vi "hmp4000_core_global.vi"() -> ()   [LabVIEW 2022 SP3]
doc: "This Global variable contains driver's:\n- Attributes\n- Range Tables\n- Repeated Capabilities"
uses:
  type_Input_Format_Attribute.ctl
  type_Input_Format_RangeTable.ctl
  type_Input_Format_RepCap.ctl
  hmp4000_rsidr_core.lvlib
panel:
  in  "Repeated Capabilities":T1[](array[typedef])=[{"repCapName"="Channel", "indetifiers"=["CH1", "CH2", "CH3", "CH4"], "cmdValues"=["1", "2", "3", "4"]}]
  in  "Range Tables":T2[](array[typedef])=[{"Type"=2, "Name"="hmp4000_rngChannel", "Entries"=[{"Name"="Not Used", "Value 1"=0.0, "Value 2"=0.0, "Command"=""}, {"Name"="Channel 1", "Value 1"=1.0, "Value 2"=0.0, "Command"="1"}, {"Name"="Channel 2", "Value 1"=2.0, "Value 2"=0.0, "Command"="2"}, {"Name"="Channel 3", "Value 1"=3.0, "Value 2"=0.0, "Command"="3"}, {"Name"="Channel 4", "Value 1"=4.0, "Value 2"=0.0, "Command"="4"}]}, {"Type"=2, "Name"="hmp4000_rngMemoryIndex", "Entries"=[{"Name"="Index 1", "Value 1"=1.0, "Value 2"=0.0, "Command"="1"}, {"Name"="Index 2", "Value 1"=2.0, "Value 2"=0.0, "Command"="2"}, {"Name"="Index 3", "Value 1"=3.0, "Value 2"=0.0, "Command"="3"}]}, {"Type"=2, "Name"="hmp4000_rngOutput", "Entries"=[{"Name"="Channel 1", "Value 1"=1.0, "Value 2"=0.0, "Command"="OUTP1"}, {"Name"="Channel 2", "Value 1"=2.0, "Value 2"=0.0, "Command"="OUTP2"}, {"Name"="Channel 3", "Value 1"=3.0, "Value 2"=0.0, "Command"="OUTP3"}, {"Name"="Channel 4", "Value 1"=4.0, "Value 2"=0.0, "Command"="OUTP4"}]}, {"Type"=0, "Name"="hmp4000_rngOutputVoltage", "Entries"=[{"Name"="", "Value 1"=0.0, "Value 2"=32.0, "Command"=""}]}, {"Type"=0, "Name"="hmp4000_rngOutputCurrent", "Entries"=[{"Name"="", "Value 1"=0.0, "Value 2"=10.0, "Command"=""}]}, {"Type"=0, "Name"="hmp4000_rngMemoryLocation", "Entries"=[{"Name"="", "Value 1"=0.0, "Value 2"=9.0, "Command"=""}]}, {"Type"=0, "Name"="hmp4000_rngArbRepetition", "Entries"=[{"Name"="", "Value 1"=0.0, "Value 2"=255.0, "Command"=""}]}, {"Type"=0, "Name"="hmp4000_rngOVP", "Entries"=[{"Name"="", "Value 1"=0.0, "Value 2"=33.0, "Command"=""}]}, {"Type"=2, "Name"="hmp4000_rngBeeper", "Entries"=[{"Name"="Off", "Value 1"=0.0, "Value 2"=0.0, "Command"="OFF"}, {"Name"="On", "Value 1"=1.0, "Value 2"=0.0, "Command"="ON"}, {"Name"="Critical Event Only", "Value 1"=2.0, "Value 2"=0.0, "Command"="CRIT"}]}, {"Type"=2, "Name"="Hmp4000_rngOverVoltageProtectionMode", "Entries"=[{"Name"="Measured", "Value 1"=0.0, "Value 2"=0.0, "Command"="MEAS"}, {"Name"="Protected", "Value 1"=1.0, "Value 2"=0.0, "Command"="PROT"}]}] {"Type" items=["Range", "Coerced", "Discrete"]}
  in  "Attributes":T3[](array[typedef])=[{"Level"=1, "Class Only"=TRUE, "Identifier"="", "Descriptive Name"="Basic Operation", "Data Type"=4, "Command"="", "Access"=0, "Range Table"="", "Read Callback"="", "Write Callback"="", "Supported Models"="", "Instrument Options"="", "Flags"=0, "Help"="This class configures Basic Operation.\n\n(1) Selection Of Channel:\nThis attribute selects the channels. \n\n(2) Output State:\nThis attribute switches On or Off the output.\n\n(3) Settings Store Location:\nThis attribute stores the settings to selected locations of a nonvolatile memory.\n\n(4) Settings Recall Location:\nThis attribute recalls the settings from selected locations of a nonvolatile memory.\n\n(5) Beeper Mode:\nThis attribute configures the beeper."}, {"Level"=2, "Class Only"=FALSE, "Identifier"="HMP4000_ATTR_SELECTION_OF_CHANNEL", "Descriptive Name"="Selection Of Channel", "Data Type"=0, "Command"="INST:SEL", "Access"=2, "Range Table"="hmp4000_rngOutput", "Read Callback"="", "Write Callback"="", "Supported Models"="", "Instrument Options"="", "Flags"=0, "Help"="This attribute selects the channels.\n\nAvailable Repeated Capabilities:\nNone\n\nRemote-control command(s):\nINSTrument:SELect"}, {"Level"=2, "Class Only"=FALSE, "Identifier"="HMP4000_ATTR_OUTPUT_STATE", "Descriptive Name"="Output State", "Data Type"=3, "Command"="OUTP:STAT", "Access"=2, "Range Table"="", "Read Callback"="", "Write Callback"="", "Supported Models"="", "Instrument Options"="", "Flags"=0, "Help"="Turns the channel output ON or OFF. When switching the channel ON, General output switch is also switched ON. When switching the channel OFF, General output switch is not changed. If changing the General output switch status is not desired, use the HMP4000_ATTR_OUTPUT_SELECT.\n\nAvailable Repeated Capabilities:\nNone\n\nRemote-control command(s):\nOUTPut:STATe"}, {"Level"=2, "Class Only"=FALSE, "Identifier"="HMP4000_ATTR_GENERAL_OUTPUT_STATE", "Descriptive Name"="General Output State", "Data Type"=3, "Command"="OUTP:GEN", "Access"=2, "Range Table"="", "Read Callback"="", "Write Callback"="", "Supported Models"="", "Instrument Options"="", "Flags"=0, "Help"="Turning on / off all previous selected channels simultaneously.\n\nAvailable Repeated Capabilities:\nNone\n\nRemote-control command(s):\nOUTPut:GENeral"}, {"Level"=2, "Class Only"=FALSE, "Identifier"="HMP4000_ATTR_OUTPUT_SELECT", "Descriptive Name"="Output Select", "Data Type"=3, "Command"="OUTP:SEL", "Access"=2, "Range Table"="", "Read Callback"="", "Write Callback"="", "Supported Models"="", "Instrument Options"="", "Flags"=0, "Help"="Activates or deactivates the previous selected channel. If the channel is activated the channel LED lights up green in CV (constant voltage) mode or red in CC (constant current) mode.\n\nAvailable Repeated Capabilities:\nNone\n\nRemote-control command(s):\nOUTPut:SELect"}, {"Level"=2, "Class Only"=FALSE, "Identifier"="HMP4000_ATTR_SETTINGS_STORE_LOCATION", "Descriptive Name"="Settings Store Location", "Data Type"=0, "Command"="*SAV", "Access"=1, "Range Table"="hmp4000_rngMemoryLocation", "Read Callback"="", "Write Callback"="", "Supported Models"="", "Instrument Options"="", "Flags"=0, "Help"="This attribute stores the settings to selected locations of a nonvolatile memory.\n\nAvailable Repeated Capabilities:\nNone\n\nRemote-control command(s):\n*SAV"}, {"Level"=2, "Class Only"=FALSE, "Identifier"="HMP4000_ATTR_SETTINGS_RECALL_LOCATION", "Descriptive Name"="Settings Recall Location", "Data Type"=0, "Command"="*RCL", "Access"=1, "Range Table"="hmp4000_rngMemoryLocation", "Read Callback"="", "Write Callback"="", "Supported Models"="", "Instrument Options"="", "Flags"=0, "Help"="This attribute recalls the settings from selected locations of a nonvolatile memory.\n\nAvailable Repeated Capabilities:\nNone\n\nRemote-control command(s):\n*RCL"}, {"Level"=2, "Class Only"=FALSE, "Identifier"="HMP4000_ATTR_BEEPER_MODE", "Descriptive Name"="Beeper Mode", "Data Type"=0, "Command"="SYST:BEEP:IMM", "Access"=2, "Range Table"="hmp4000_rngBeeper", "Read Callback"="", "Write Callback"="", "Supported Models"="", "Instrument Options"="", "Flags"=0, "Help"="This attribute configures the beeper.\n\nAvailable Repeated Capabilities:\nNone\n\nRemote-control command(s):\nSYSTem:BEEPer:IMMediate"}, {"Level"=1, "Class Only"=TRUE, "Identifier"="", "Descriptive Name"="Voltage and Current", "Data Type"=4, "Command"="", "Access"=0, "Range Table"="", "Read Callback"="", "Write Callback"="", "Supported Models"="", "Instrument Options"="", "Flags"=0, "Help"="This class configures Voltage and Current.\n\n(1) Output Voltage Level:\nThis attribute adjusts the output voltage level. \n\n(2) Output Voltage Level Step:\nThis attribute configures the output voltage step value. \n\n(3) Over Voltage Protection Level:\nThis attribute configures the over voltage protection (OVP). \n\n(4) Query Over Voltage Protection Status:\nThis attribute queries the over voltage protection (OVP) status. \n\n(5) Over Voltage Protection Clear:\nThis attribute clears the over voltage protection (OVP). \n\n(6) Output Current Level:\nThis attribute adjusts the output current level. \n\n(7) Output Current Level Step:\nThis attribute configures the output current step value. \n\n(8) Electronic Fuse State:\nThis attribute switches On or Off the electronic fuse.\n\n(9) Query Electronic Fuse Status:\nThis attribute queries the electronic fuse status. \n\n(10) Electronic Fuse Channel Link:\nThis attribute link electronic fuse to the channel.\n\n(11) Electronic Fuse Channel Unlink:\nThis attribute unlink electronic fuse from the channel."}, {"Level"=2, "Class Only"=FALSE, "Identifier"="HMP4000_ATTR_OUTPUT_VOLTAGE_LEVEL", "Descriptive Name"="Output Voltage Level", "Data Type"=1, "Command"="SOUR:VOLT:LEV:AMPL", "Access"=2, "Range Table"="hmp4000_rngOutputVoltage", "Read Callback"="", "Write Callback"="", "Supported Models"="", "Instrument Options"="", "Flags"=0, "Help"="This attribute adjusts the output voltage level.\n\nAvailable Repeated Capabilities:\nNone\n\nRemote-control command(s):\nSOURce:VOLTage:LEVel:AMPLitude"}, {"Level"=2, "Class Only"=FALSE, "Identifier"="HMP4000_ATTR_OUTPUT_VOLTAGE_LEVEL_MAX", "Descriptive Name"="Output Voltage Level Max", "Data Type"=1, "Command"="VOLT? MAX", "Access"=0, "Range Table"="", "Read Callback"="", "Write Callback"="", "Supported Models"="", "Instrument Options"="", "Flags"=0, "Help"="Queires the maximum available output voltage.\n\nAvailable Repeated Capabilities:\nNone\n\nRemote-control command(s):\n[SOURce:]VOLTage[:LEVel][:IMMediate][:AMPLitude]"}, {"Level"=2, "Class Only"=FALSE, "Identifier"="HMP4000_ATTR_OUTPUT_VOLTAGE_LEVEL_STEP", "Descriptive Name"="Output Voltage Level Step", "Data Type"=1, "Command"="SOUR:VOLT:LEV:AMPL:STEP:INCR", "Access"=2, "Range Table"="hmp4000_rngOutputVoltage", "Read Callback"="", "Write Callback"="", "Supported Models"="", "Instrument Options"="", "Flags"=0, "Help"="This attribute configures the output voltage step value.\n\nAvailable Repeated Capabilities:\nNone\n\nRemote-control command(s):\nSOURce:VOLTage:LEVel:AMPLitude:STEP:INCRement"}, {"Level"=2, "Class Only"=FALSE, "Identifier"="HMP4000_ATTR_OVER_VOLTAGE_PROTECTION_LEVEL", "Descriptive Name"="Over Voltage Protection Level", "Data Type"=1, "Command"="VOLT:PROT:LEV", "Access"=2, "Range Table"="hmp4000_rngOVP", "Read Callback"="", "Write Callback"="", "Supported Models"="", "Instrument Options"="", "Flags"=0, "Help"="This attribute configures the over voltage protection (OVP).\n\nAvailable Repeated Capabilities:\nNone\n\nRemote-control command(s):\nVOLTage:PROTection:LEVel"}, {"Level"=2, "Class Only"=FALSE, "Identifier"="HMP4000_ATTR_QUERY_OVER_VOLTAGE_PROTECTION_STATUS", "Descriptive Name"="Query Over Voltage Protection Status", "Data Type"=3, "Command"="VOLT:PROT:TRIP?", "Access"=0, "Range Table"="", "Read Callback"="", "Write Callback"="", "Supported Models"="", "Instrument Options"="", "Flags"=0, "Help"="This attribute queries the over voltage protection (OVP) status.\n\nAvailable Repeated Capabilities:\nNone\n\nRemote-control command(s):\nVOLTage:PROTection:TRIPped?"}, {"Level"=2, "Class Only"=FALSE, "Identifier"="HMP4000_ATTR_OVER_VOLTAGE_PROTECTION_CLEAR", "Descriptive Name"="Over Voltage Protection Clear", "Data Type"=4, "Command"="VOLT:PROT:CLE", "Access"=1, "Range Table"="", "Read Callback"="", "Write Callback"="", "Supported Models"="", "Instrument Options"="", "Flags"=0, "Help"="This attribute clears the over voltage protection (OVP).\n\nAvailable Repeated Capabilities:\nNone\n\nRemote-control command(s):\nVOLTage:PROTection:CLEar"}, {"Level"=2, "Class Only"=FALSE, "Identifier"="HMP4000_ATTR_OVER_VOLTAGE_PROTECTION_MODE", "Descriptive Name"="Over Voltage Protection Mode", "Data Type"=0, "Command"="VOLT:PROT:MODE", "Access"=2, "Range Table"="Hmp4000_rngOverVoltageProtectionMode", "Read Callback"="", "Write Callback"="", "Supported Models"="", "Instrument Options"="", "Flags"=0, "Help"="Sets the OVP mode for the previously selected channel.\n\nAvailable Repeated Capabilities:\nNone\n\nRemote-control command(s):\n[SOURce:]VOLTage:PROTection:MODE"}, {"Level"=2, "Class Only"=FALSE, "Identifier"="HMP4000_ATTR_OUTPUT_CURRENT_LEVEL", "Descriptive Name"="Output Current Level", "Data Type"=1, "Command"="SOUR:CURR:LEV:AMPL", "Access"=2, "Range Table"="hmp4000_rngOutputCurrent", "Read Callback"="", "Write Callback"="", "Supported Models"="", "Instrument Options"="", "Flags"=0, "Help"="This attribute adjusts the output current level.\n\nAvailable Repeated Capabilities:\nNone\n\nRemote-control command(s):\nSOURce:CURRent:LEVel:AMPLitude"}, {"Level"=2, "Class Only"=FALSE, "Identifier"="HMP4000_ATTR_OUTPUT_CURRENT_LEVEL_MAX", "Descriptive Name"="Output Current Level Max", "Data Type"=1, "Command"="CURR? MAX", "Access"=0, "Range Table"="", "Read Callback"="", "Write Callback"="", "Supported Models"="", "Instrument Options"="", "Flags"=0, "Help"="Queries the maximum allowed current value.\n\nAvailable Repeated Capabilities:\nNone\n\nRemote-control command(s):\n[SOURce:]CURRent[:LEVel][:IMMediate][:AMPLitude]"}, {"Level"=2, "Class Only"=FALSE, "Identifier"="HMP4000_ATTR_OUTPUT_CURRENT_LEVEL_STEP", "Descriptive Name"="Output Current Level Step", "Data Type"=1, "Command"="SOUR:CURR:LEV:AMPL:STEP:INCR", "Access"=2, "Range Table"="hmp4000_rngOutputCurrent", "Read Callback"="", "Write Callback"="", "Supported Models"="", "Instrument Options"="", "Flags"=0, "Help"="This attribute configures the output current step value.\n\nAvailable Repeated Capabilities:\nNone\n\nRemote-control command(s):\nSOURce:CURRent:LEVel:AMPLitude:STEP:INCRement"}, {"Level"=2, "Class Only"=FALSE, "Identifier"="HMP4000_ATTR_ELECTRONIC_FUSE_STATE", "Descriptive Name"="Electronic Fuse State", "Data Type"=3, "Command"="FUSE:STAT", "Access"=2, "Range Table"="", "Read Callback"="", "Write Callback"="", "Supported Models"="", "Instrument Options"="", "Flags"=0, "Help"="This attribute switches On or Off the electronic fuse.\n\nAvailable Repeated Capabilities:\nNone\n\nRemote-control command(s):\nFUSE:STATe"}, {"Level"=2, "Class Only"=FALSE, "Identifier"="HMP4000_ATTR_QUERY_ELECTRONIC_FUSE_STATUS", "Descriptive Name"="Query Electronic Fuse Status", "Data Type"=3, "Command"="FUSE:TRIP?", "Access"=0, "Range Table"="", "Read Callback"="", "Write Callback"="", "Supported Models"="", "Instrument Options"="", "Flags"=0, "Help"="This attribute queries the electronic fuse status.\n\nAvailable Repeated Capabilities:\nNone\n\nRemote-control command(s):\nFUSE:TRIPped?"}, {"Level"=2, "Class Only"=FALSE, "Identifier"="HMP4000_ATTR_ELECTRONIC_FUSE_CHANNEL_LINK", "Descriptive Name"="Electronic Fuse Channel Link", "Data Type"=0, "Command"="FUSE:LINK", "Access"=1, "Range Table"="hmp4000_rngChannel", "Read Callback"="", "Write Callback"="", "Supported Models"="", "Instrument Options"="", "Flags"=0, "Help"="This attribute link electronic fuse to the channel.\n\nAvailable Repeated Capabilities:\nNone\n\nRemote-control command(s):\nFUSE:LINK"}, {"Level"=2, "Class Only"=FALSE, "Identifier"="HMP4000_ATTR_ELECTRONIC_FUSE_CHANNEL_UNLINK", "Descriptive Name"="Electronic Fuse Channel Unlink", "Data Type"=0, "Command"="FUSE:UNL", "Access"=1, "Range Table"="hmp4000_rngChannel", "Read Callback"="", "Write Callback"="", "Supported Models"="", "Instrument Options"="", "Flags"=0, "Help"="This attribute unlink electronic fuse from the channel.\n\nAvailable Repeated Capabilities:\nNone\n\nRemote-control command(s):\nFUSE:UNLink"}, {"Level"=2, "Class Only"=TRUE, "Identifier"="", "Descriptive Name"="Query Combined Voltage And Current", "Data Type"=4, "Command"="", "Access"=0, "Range Table"="", "Read Callback"="", "Write Callback"="", "Supported Models"="", "Instrument Options"="", "Flags"=0, "Help"="This function queries combined setting of voltage and current. \n\nFirst result is Voltage Value, second is Current.\n\nRemote-control command(s):\nAPPLy?"}, {"Level"=1, "Class Only"=TRUE, "Identifier"="", "Descriptive Name"="Arbitrary Generator", "Data Type"=4, "Command"="", "Access"=0, "Range Table"="", "Read Callback"="", "Write Callback"="", "Supported Models"="", "Instrument Options"="", "Flags"=0, "Help"="This class configures Arbitrary Generator.\n\n(1) Arbitrary Generator Repetition:\nNo. of repetition. The maximum number of repetitions is 255. If 0 is selected, the waveform will be repeated indefi nitely.\n\n(2) Arbitrary Generator Start Channel:\nThis attribute selects the channel for starting arbitrary generator. \n\n(3) Arbitrary Generator Stop Channel:\nThis attribute selects the channel for stoping arbitrary generator. \n\n(4) Arbitrary Generator Data Transfer Channel:\nThis attribute selects the channel where the data entered are sent to.\n\n(5) Arbitrary Generator Save:\nThis attribute selects the storage for saving arbitrary generator waveform data. \n\n\n(6) Arbitrary Generator Recall:\nThis attribute selects the storage for recalling arbitrary generator waveform data. \n\n(7) Arbitrary Generator Clear:\nThis attribute selects the storage for clearing arbitrary generator waveform data."}, {"Level"=2, "Class Only"=TRUE, "Identifier"="", "Descriptive Name"="Configure Arbitrary Generator Waveform Data", "Data Type"=4, "Command"="", "Access"=0, "Range Table"="", "Read Callback"="", "Write Callback"="", "Supported Models"="", "Instrument Options"="", "Flags"=0, "Help"="This function sets the parameters of the freely programmable waveforms. Set points defining voltage, current and dwell\ntime are required.\n\nA maximum of 128 set points (index 0 ... 128) may be used and\nwill be repetitively addressed.\n\nThe maximum number of repetitions is 255. If Repetitons 0 is selected, the waveform will be repeated indefinitely. \n\nRemote-control command(s):\nARBitrary:DATA <voltage1, current1, time1, voltage2, ...>"}, {"Level"=2, "Class Only"=FALSE, "Identifier"="HMP4000_ATTR_ARBITRARY_GENERATOR_REPETITION", "Descriptive Name"="Arbitrary Generator Repetition", "Data Type"=0, "Command"="ARB:REP", "Access"=2, "Range Table"="hmp4000_rngArbRepetition", "Read Callback"="", "Write Callback"="", "Supported Models"="", "Instrument Options"="", "Flags"=0, "Help"="No. of repetition. The maximum number of repetitions is 255. If 0 is selected, the waveform will be repeated indefi nitely.\n\nAvailable Repeated Capabilities:\nNone\n\nRemote-control command(s):\nARBitrary:REPetitions"}, {"Level"=2, "Class Only"=FALSE, "Identifier"="HMP4000_ATTR_ARBITRARY_GENERATOR_START_CHANNEL", "Descriptive Name"="Arbitrary Generator Start Channel", "Data Type"=0, "Command"="ARB:STAR", "Access"=1, "Range Table"="hmp4000_rngChannel", "Read Callback"="", "Write Callback"="", "Supported Models"="", "Instrument Options"="", "Flags"=0, "Help"="This attribute selects the channel for starting arbitrary generator.\n\nAvailable Repeated Capabilities:\nNone\n\nRemote-control command(s):\nARBitrary:STARt"}, {"Level"=2, "Class Only"=FALSE, "Identifier"="HMP4000_ATTR_ARBITRARY_GENERATOR_STOP_CHANNEL", "Descriptive Name"="Arbitrary Generator Stop Channel", "Data Type"=0, "Command"="ARB:STOP", "Access"=1, "Range Table"="hmp4000_rngChannel", "Read Callback"="", "Write Callback"="", "Supported Models"="", "Instrument Options"="", "Flags"=0, "Help"="This attribute selects the channel for stoping arbitrary generator.\n\nAvailable Repeated Capabilities:\nNone\n\nRemote-control command(s):\nARBitrary:STOP"}, {"Level"=2, "Class Only"=FALSE, "Identifier"="HMP4000_ATTR_ARBITRARY_GENERATOR_DATA_TRANSFER_CHANNEL", "Descriptive Name"="Arbitrary Generator Data Transfer Channel", "Data Type"=0, "Command"="ARB:TRAN", "Access"=1, "Range Table"="hmp4000_rngChannel", "Read Callback"="", "Write Callback"="", "Supported Models"="", "Instrument Options"="", "Flags"=0, "Help"="This attribute selects the channel where the data entered are sent to.\n\nAvailable Repeated Capabilities:\nNone\n\nRemote-control command(s):\nARBitrary:TRANsfer"}, {"Level"=2, "Class Only"=FALSE, "Identifier"="HMP4000_ATTR_ARBITRARY_GENERATOR_SAVE", "Descriptive Name"="Arbitrary Generator Save", "Data Type"=0, "Command"="ARB:SAVE", "Access"=1, "Range Table"="hmp4000_rngMemoryIndex", "Read Callback"="", "Write Callback"="hmp4000_Delayed_Int32_WriteCallback.vi", "Supported Models"="", "Instrument Options"="", "Flags"=0, "Help"="This attribute selects the storage for saving arbitrary generator waveform data.\n\nAvailable Repeated Capabilities:\nNone\n\nRemote-control command(s):\nARBitrary:SAVE"}, {"Level"=2, "Class Only"=FALSE, "Identifier"="HMP4000_ATTR_ARBITRARY_GENERATOR_RECALL", "Descriptive Name"="Arbitrary Generator Recall", "Data Type"=0, "Command"="ARB:REST", "Access"=1, "Range Table"="hmp4000_rngMemoryIndex", "Read Callback"="", "Write Callback"="", "Supported Models"="", "Instrument Options"="", "Flags"=0, "Help"="This attribute selects the storage for recalling arbitrary generator waveform data.\n\nAvailable Repeated Capabilities:\nNone\n\nRemote-control command(s):\nARBitrary:RESTore"}, {"Level"=2, "Class Only"=FALSE, "Identifier"="HMP4000_ATTR_ARBITRARY_GENERATOR_CLEAR", "Descriptive Name"="Arbitrary Generator Clear", "Data Type"=0, "Command"="ARB:CLE", "Access"=1, "Range Table"="hmp4000_rngMemoryIndex", "Read Callback"="", "Write Callback"="", "Supported Models"="", "Instrument Options"="", "Flags"=0, "Help"="This attribute selects the storage for clearing arbitrary generator waveform data.\n\nAvailable Repeated Capabilities:\nNone\n\nRemote-control command(s):\nARBitrary:CLEar"}, {"Level"=1, "Class Only"=TRUE, "Identifier"="", "Descriptive Name"="Measurement", "Data Type"=4, "Command"="", "Access"=0, "Range Table"="", "Read Callback"="", "Write Callback"="", "Supported Models"="", "Instrument Options"="", "Flags"=0, "Help"="This class queries measurement.\n\n(1) Measurement DC Voltage:\nThis attribute queries the measured voltage value. \n\n(2) Measurement DC Current:\nThis attribute queries the measured Current value."}, {"Level"=2, "Class Only"=FALSE, "Identifier"="HMP4000_ATTR_MEASUREMENT_DC_VOLTAGE", "Descriptive Name"="Measurement DC Voltage", "Data Type"=1, "Command"="MEAS:VOLT:DC?", "Access"=0, "Range Table"="", "Read Callback"="", "Write Callback"="", "Supported Models"="", "Instrument Options"="", "Flags"=0, "Help"="This attribute queries the measured voltage value.\n\nAvailable Repeated Capabilities:\nNone\n\nRemote-control command(s):\nMEASure:VOLTage:DC?"}, {"Level"=2, "Class Only"=FALSE, "Identifier"="HMP4000_ATTR_MEASUREMENT_DC_CURRENT", "Descriptive Name"="Measurement DC Current", "Data Type"=1, "Command"="MEAS:CURR:DC?", "Access"=0, "Range Table"="", "Read Callback"="", "Write Callback"="", "Supported Models"="", "Instrument Options"="", "Flags"=0, "Help"="This attribute queries the measured Current value.\n\nAvailable Repeated Capabilities:\nNone\n\nRemote-control command(s):\nMEASure:CURRent:DC?"}, {"Level"=1, "Class Only"=TRUE, "Identifier"="", "Descriptive Name"="Utility Functions", "Data Type"=4, "Command"="", "Access"=0, "Range Table"="", "Read Callback"="", "Write Callback"="", "Supported Models"="", "Instrument Options"="", "Flags"=0, "Help"="Various utility attributes.\n\n(1) System Version:\nGets system version.\n\n(2) System Error:\nThis attribute queries the earliest entry in the error queue, and deletes it after the readout.\n\n(3) System All Errors:\nReads all errors from instrument.\n\n(4) Questionable Enable Register:\nThis attribute configures the selected register enable values.\n\n(5) Questionable Instrument Enable Register:\nThis attribute configures the selected register enable values.\n\n(6) Questionable Instrument Specific Enable Register:\nThis attribute configures the selected register enable values.\n\n(7) Questionable Instrument Specific Condition Register:\nThis attribute queries the selected register condition values."}, {"Level"=2, "Class Only"=TRUE, "Identifier"="", "Descriptive Name"="Add Stream Logger", "Data Type"=4, "Command"="", "Access"=0, "Range Table"="", "Read Callback"="", "Write Callback"="", "Supported Models"="", "Instrument Options"="", "Flags"=0, "Help"="This method adds the stream for logging."}, {"Level"=2, "Class Only"=TRUE, "Identifier"="", "Descriptive Name"="Remove Stream Logger", "Data Type"=4, "Command"="", "Access"=0, "Range Table"="", "Read Callback"="", "Write Callback"="", "Supported Models"="", "Instrument Options"="", "Flags"=0, "Help"="This method removes the stream for logging."}, {"Level"=2, "Class Only"=TRUE, "Identifier"="", "Descriptive Name"="Write String To Log", "Data Type"=4, "Command"="", "Access"=0, "Range Table"="", "Read Callback"="", "Write Callback"="", "Supported Models"="", "Instrument Options"="", "Flags"=0, "Help"="Writes string message to log."}, {"Level"=2, "Class Only"=TRUE, "Identifier"="", "Descriptive Name"="Read To File From Instrument", "Data Type"=4, "Command"="", "Access"=0, "Range Table"="", "Read Callback"="", "Write Callback"="", "Supported Models"="", "Instrument Options"="", "Flags"=0, "Help"="Is used to read data from the instrument and write it to a user specified file on the host computer.\n\nRemote-control command(s):\nMMEMory:DATA? <file_name>"}, {"Level"=2, "Class Only"=TRUE, "Identifier"="", "Descriptive Name"="Write From File To Instrument", "Data Type"=4, "Command"="", "Access"=0, "Range Table"="", "Read Callback"="", "Write Callback"="", "Supported Models"="", "Instrument Options"="", "Flags"=0, "Help"="Is used to read data from the host computer and write it to a user specified file in the instrument.\n\nRemote-control command(s):\nMMEMory:DATA <file_name>"}, {"Level"=2, "Class Only"=TRUE, "Identifier"="", "Descriptive Name"="Query Binary Data Block To Stream", "Data Type"=4, "Command"="", "Access"=0, "Range Table"="", "Read Callback"="", "Write Callback"="", "Supported Models"="", "Instrument Options"="", "Flags"=0, "Help"="Queries IEEE binary data block from instrument to stream. Use it for fast fetching of binary block data."}, {"Level"=2, "Class Only"=TRUE, "Identifier"="", "Descriptive Name"="Query Binary Data Block To Stream With OPC", "Data Type"=4, "Command"="", "Access"=0, "Range Table"="", "Read Callback"="", "Write Callback"="", "Supported Models"="", "Instrument Options"="", "Flags"=0, "Help"="Queries IEEE binary data block from instrument to stream. Use it for fast fetching of binary block data. If timeout is null, -1 or 0, the current Opc Timeout is used."}, {"Level"=2, "Class Only"=TRUE, "Identifier"="", "Descriptive Name"="Write Binary Block From Stream", "Data Type"=4, "Command"="", "Access"=0, "Range Table"="", "Read Callback"="", "Write Callback"="", "Supported Models"="", "Instrument Options"="", "Flags"=0, "Help"="Writes IEEE binary data block from stream to instrument. You need to specify the SCPI command to prepend the binary data block."}, {"Level"=2, "Class Only"=TRUE, "Identifier"="", "Descriptive Name"="Query Bool", "Data Type"=4, "Command"="", "Access"=0, "Range Table"="", "Read Callback"="", "Write Callback"="", "Supported Models"="", "Instrument Options"="", "Flags"=0, "Help"="This method queries the bool value."}, {"Level"=2, "Class Only"=TRUE, "Identifier"="", "Descriptive Name"="Query Int32", "Data Type"=4, "Command"="", "Access"=0, "Range Table"="", "Read Callback"="", "Write Callback"="", "Supported Models"="", "Instrument Options"="", "Flags"=0, "Help"="This method queries the int32 value."}, {"Level"=2, "Class Only"=TRUE, "Identifier"="", "Descriptive Name"="Query Double", "Data Type"=4, "Command"="", "Access"=0, "Range Table"="", "Read Callback"="", "Write Callback"="", "Supported Models"="", "Instrument Options"="", "Flags"=0, "Help"="This method queries the double value."}, {"Level"=2, "Class Only"=TRUE, "Identifier"="", "Descriptive Name"="Query String", "Data Type"=4, "Command"="", "Access"=0, "Range Table"="", "Read Callback"="", "Write Callback"="", "Supported Models"="", "Instrument Options"="", "Flags"=0, "Help"="This method queries the string value."}, {"Level"=2, "Class Only"=TRUE, "Identifier"="", "Descriptive Name"="Write Command with OPC sync", "Data Type"=4, "Command"="", "Access"=0, "Range Table"="", "Read Callback"="", "Write Callback"="", "Supported Models"="", "Instrument Options"="", "Flags"=0, "Help"="Sends a command to the instrument synchronised with OPC-polling. Use this function to wait for an instrument operation that can take a long time to complete, e.g. self-alignment. If timeout is null, -1 or 0, the current Opc Timeout is used."}, {"Level"=2, "Class Only"=TRUE, "Identifier"="", "Descriptive Name"="Query with OPC sync", "Data Type"=4, "Command"="", "Access"=0, "Range Table"="", "Read Callback"="", "Write Callback"="", "Supported Models"="", "Instrument Options"="", "Flags"=0, "Help"="Sends a query to the instrument synchronised with OPC-polling. Use this function to wait for a response that can take a long time to complete e.g. self-alignment, calibration or self-test. If timeout is null, -1 or 0, the current Opc Timeout is used."}, {"Level"=2, "Class Only"=TRUE, "Identifier"="", "Descriptive Name"="Self Test", "Data Type"=4, "Command"="", "Access"=0, "Range Table"="", "Read Callback"="", "Write Callback"="", "Supported Models"="", "Instrument Options"="", "Flags"=0, "Help"="Runs the instrument's self test routine."}, {"Level"=2, "Class Only"=TRUE, "Identifier"="", "Descriptive Name"="Revision Query", "Data Type"=4, "Command"="", "Access"=0, "Range Table"="", "Read Callback"="", "Write Callback"="", "Supported Models"="", "Instrument Options"="", "Flags"=0, "Help"="Returns the revision numbers of the instrument driver and instrument firmware, and tells the user with which  instrument firmware this revision of the driver is compatible."}, {"Level"=2, "Class Only"=TRUE, "Identifier"="", "Descriptive Name"="Delay", "Data Type"=4, "Command"="", "Access"=0, "Range Table"="", "Read Callback"="", "Write Callback"="", "Supported Models"="", "Instrument Options"="", "Flags"=0, "Help"="Suspends the program for the selected number of second."}, {"Level"=2, "Class Only"=TRUE, "Identifier"="", "Descriptive Name"="Error Query All", "Data Type"=4, "Command"="", "Access"=0, "Range Table"="", "Read Callback"="", "Write Callback"="", "Supported Models"="", "Instrument Options"="", "Flags"=0, "Help"="Returns all error.\n\nRemote-control command(s):\nSYSTem:ERRor?"}, {"Level"=2, "Class Only"=TRUE, "Identifier"="", "Descriptive Name"="Get Instrument Options", "Data Type"=4, "Command"="", "Access"=0, "Range Table"="", "Read Callback"="", "Write Callback"="", "Supported Models"="", "Instrument Options"="", "Flags"=0, "Help"="Returns all the instrument options.\n\nRemote-control command(s):\n*OPT?"}, {"Level"=2, "Class Only"=TRUE, "Identifier"="", "Descriptive Name"="Read Bytes", "Data Type"=4, "Command"="", "Access"=0, "Range Table"="", "Read Callback"="", "Write Callback"="", "Supported Models"="", "Instrument Options"="", "Flags"=0, "Help"="Reads a complete response from the instrument."}, {"Level"=2, "Class Only"=TRUE, "Identifier"="", "Descriptive Name"="Read String", "Data Type"=4, "Command"="", "Access"=0, "Range Table"="", "Read Callback"="", "Write Callback"="", "Supported Models"="", "Instrument Options"="", "Flags"=0, "Help"="Reads a complete response from the instrument and returns it as a string."}, {"Level"=2, "Class Only"=TRUE, "Identifier"="", "Descriptive Name"="Write Bytes", "Data Type"=4, "Command"="", "Access"=0, "Range Table"="", "Read Callback"="", "Write Callback"="", "Supported Models"="", "Instrument Options"="", "Flags"=0, "Help"="Write an array of bytes to the device."}, {"Level"=2, "Class Only"=TRUE, "Identifier"="", "Descriptive Name"="Write String", "Data Type"=4, "Command"="", "Access"=0, "Range Table"="", "Read Callback"="", "Write Callback"="", "Supported Models"="", "Instrument Options"="", "Flags"=0, "Help"="Write a string to the device."}, {"Level"=2, "Class Only"=FALSE, "Identifier"="HMP4000_ATTR_SYSTEM_VERSION", "Descriptive Name"="System Version", "Data Type"=2, "Command"="SYST:VERSion?", "Access"=0, "Range Table"="", "Read Callback"="", "Write Callback"="", "Supported Models"="", "Instrument Options"="", "Flags"=0, "Help"="Gets system version.\n\nAvailable Repeated Capabilities:\nNone\n\nRemote-control command(s):\nSYSTem:VERSion?"}, {"Level"=2, "Class Only"=FALSE, "Identifier"="HMP4000_ATTR_SYSTEM_ERROR", "Descriptive Name"="System Error", "Data Type"=2, "Command"="SYST:ERRor?", "Access"=0, "Range Table"="", "Read Callback"="", "Write Callback"="", "Supported Models"="", "Instrument Options"="", "Flags"=0, "Help"="This attribute queries the earliest entry in the error queue, and deletes it after the readout.\n\nAvailable Repeated Capabilities:\nNone\n\nRemote-control command(s):\nSYSTem:ERRor?"}, {"Level"=2, "Class Only"=FALSE, "Identifier"="HMP4000_ATTR_SYSTEM_ALL_ERRORS", "Descriptive Name"="System All Errors", "Data Type"=2, "Command"="SYST:ERR:ALL?", "Access"=0, "Range Table"="", "Read Callback"="", "Write Callback"="", "Supported Models"="", "Instrument Options"="", "Flags"=0, "Help"="Reads all errors from instrument.\n\nAvailable Repeated Capabilities:\nNone\n\nRemote-control command(s):\nSYSTem:ERRor:ALL?"}, {"Level"=2, "Class Only"=FALSE, "Identifier"="HMP4000_ATTR_SYSTEM_LOCAL", "Descriptive Name"="System Local", "Data Type"=4, "Command"="SYST:LOC", "Access"=1, "Range Table"="", "Read Callback"="", "Write Callback"="", "Supported Models"="", "Instrument Options"="", "Flags"=2, "Help"="Sets the system to front panel control. The front panel control is unlocked.\n\nAvailable Repeated Capabilities:\nNone\n\nRemote-control command(s):\nSYSTem:LOCal"}, {"Level"=2, "Class Only"=FALSE, "Identifier"="HMP4000_ATTR_SYSTEM_REMOTE", "Descriptive Name"="System Remote", "Data Type"=4, "Command"="SYST:REM", "Access"=1, "Range Table"="", "Read Callback"="", "Write Callback"="", "Supported Models"="", "Instrument Options"="", "Flags"=2, "Help"="Sets the system to remote state. The front panel control is locked. By pushing the REMOTE button the front panel control will be activated. If the instrument receives a remote command it will be switched into remote control automatically (REMOTE button LED lights up).\n\nAvailable Repeated Capabilities:\nNone\n\nRemote-control command(s):\nSYSTem:REMote"}, {"Level"=2, "Class Only"=FALSE, "Identifier"="HMP4000_ATTR_SYSTEM_REMOTE_LOCK", "Descriptive Name"="System Remote Lock", "Data Type"=4, "Command"="SYST:RWL", "Access"=1, "Range Table"="", "Read Callback"="", "Write Callback"="", "Supported Models"="", "Instrument Options"="", "Flags"=2, "Help"="Sets the system to remote state. The front panel control is locked and can not be unlocked via REMOTE button). You are only able to unlock the front panel control via SCPI command SYSTem:LOCal.\n\nAvailable Repeated Capabilities:\nNone\n\nRemote-control command(s):\nSYSTem:RWLock"}, {"Level"=2, "Class Only"=FALSE, "Identifier"="HMP4000_ATTR_SYSTEM_REMOTE_MIX", "Descriptive Name"="System Remote Mix", "Data Type"=4, "Command"="SYST:MIX", "Access"=1, "Range Table"="", "Read Callback"="", "Write Callback"="", "Supported Models"="", "Instrument Options"="", "Flags"=2, "Help"="Sets the system to remote state. The front panel and remote control are possible simultaneously (mixed mode).\n\nAvailable Repeated Capabilities:\nNone\n\nRemote-control command(s):\nSYSTem:MIX"}, {"Level"=2, "Class Only"=FALSE, "Identifier"="HMP4000_ATTR_QUESTIONABLE_ENABLE_REGISTER", "Descriptive Name"="Questionable Enable Register", "Data Type"=0, "Command"="STAT:QUES:ENAB", "Access"=2, "Range Table"="", "Read Callback"="", "Write Callback"="", "Supported Models"="", "Instrument Options"="", "Flags"=0, "Help"="This attribute configures the selected register enable values.\n\nAvailable Repeated Capabilities:\nNone\n\nRemote-control command(s):\nSTATus:QUEStionable:ENABle"}, {"Level"=2, "Class Only"=FALSE, "Identifier"="HMP4000_ATTR_QUESTIONABLE_INSTRUMENT_ENABLE_REGISTER", "Descriptive Name"="Questionable Instrument Enable Register", "Data Type"=0, "Command"="STAT:QUES:INST:ENAB", "Access"=2, "Range Table"="", "Read Callback"="", "Write Callback"="", "Supported Models"="", "Instrument Options"="", "Flags"=0, "Help"="This attribute configures the selected register enable values.\n\nAvailable Repeated Capabilities:\nNone\n\nRemote-control command(s):\nSTATus:QUEStionable:INSTrument:ENABle"}, {"Level"=2, "Class Only"=FALSE, "Identifier"="HMP4000_ATTR_ID_QUERY_RESPONSE", "Descriptive Name"="ID Query Response", "Data Type"=2, "Command"="*IDN?", "Access"=0, "Range Table"="", "Read Callback"="", "Write Callback"="", "Supported Models"="", "Instrument Options"="", "Flags"=0, "Help"="Returns the ID Query response string. The instrument driver gets the value of this attribute when you pass VI_TRUE for the ID Query parameter to the hmp4000_init or hmp4000_InitWithOptions function.\n\nAvailable Repeated Capabilities:\nNone\n\nRemote-control command(s):\n*IDN?"}, {"Level"=2, "Class Only"=TRUE, "Identifier"="", "Descriptive Name"="Reset", "Data Type"=4, "Command"="", "Access"=0, "Range Table"="", "Read Callback"="", "Write Callback"="", "Supported Models"="", "Instrument Options"="", "Flags"=0, "Help"="This function resets the instrument to a known state and sends initialization commands to the instrument. The initialization commands set instrument settings such as Headers Off, Short Command form, and Data Transfer Binary to the state necessary for the operation of the instrument driver.\n\nRemote-control command(s):\n*RST"}, {"Level"=2, "Class Only"=TRUE, "Identifier"="", "Descriptive Name"="Clear Status", "Data Type"=4, "Command"="", "Access"=0, "Range Table"="", "Read Callback"="", "Write Callback"="", "Supported Models"="", "Instrument Options"="", "Flags"=0, "Help"="This function clears status.\n\nRemote-control command(s):\n*CLS"}, {"Level"=2, "Class Only"=TRUE, "Identifier"="", "Descriptive Name"="Channel", "Data Type"=4, "Command"="", "Access"=0, "Range Table"="", "Read Callback"="", "Write Callback"="", "Supported Models"="", "Instrument Options"="", "Flags"=0, "Help"="Contains settings for channel."}, {"Level"=3, "Class Only"=FALSE, "Identifier"="HMP4000_ATTR_QUESTIONABLE_INSTRUMENT_SPECIFIC_ENABLE_REGISTER", "Descriptive Name"="Questionable Instrument Specific Enable Register", "Data Type"=0, "Command"="STAT:QUES:INST:ISUM{Channel}:ENAB", "Access"=2, "Range Table"="", "Read Callback"="", "Write Callback"="", "Supported Models"="", "Instrument Options"="", "Flags"=0, "Help"="This attribute configures the selected register enable values.\n\nAvailable Repeated Capabilities:\nChannel: CH1,CH2,CH3,CH4\r\n\nRemote-control command(s):\nSTATus:QUEStionable:INSTrument:ISUMmary<channel>:ENABle"}, {"Level"=3, "Class Only"=FALSE, "Identifier"="HMP4000_ATTR_QUESTIONABLE_INSTRUMENT_SPECIFIC_CONDITION_REGISTER", "Descriptive Name"="Questionable Instrument Specific Condition Register", "Data Type"=0, "Command"="STAT:QUES:INST:ISUM{Channel}:COND?", "Access"=0, "Range Table"="", "Read Callback"="", "Write Callback"="", "Supported Models"="", "Instrument Options"="", "Flags"=0, "Help"="This attribute queries the selected register condition values.\n\nAvailable Repeated Capabilities:\nChannel: CH1,CH2,CH3,CH4\r\n\nRemote-control command(s):\nSTATus:QUEStionable:INSTrument:ISUMmary<channel>:CONDition?"}] {"Flags" format="%08b"; "Access" items=["Read Only", "Write Only", "Read/Write"]; "Data Type" items=["Integer 32", "Double", "String", "Boolean", "None", "Integer 64", "RawString"]}
  in  "Supported Models":string[](array[string])=["HMP4000", "HMP4030", "HMP4040", "HMP2000", "HMP2020", "HMP2030"]
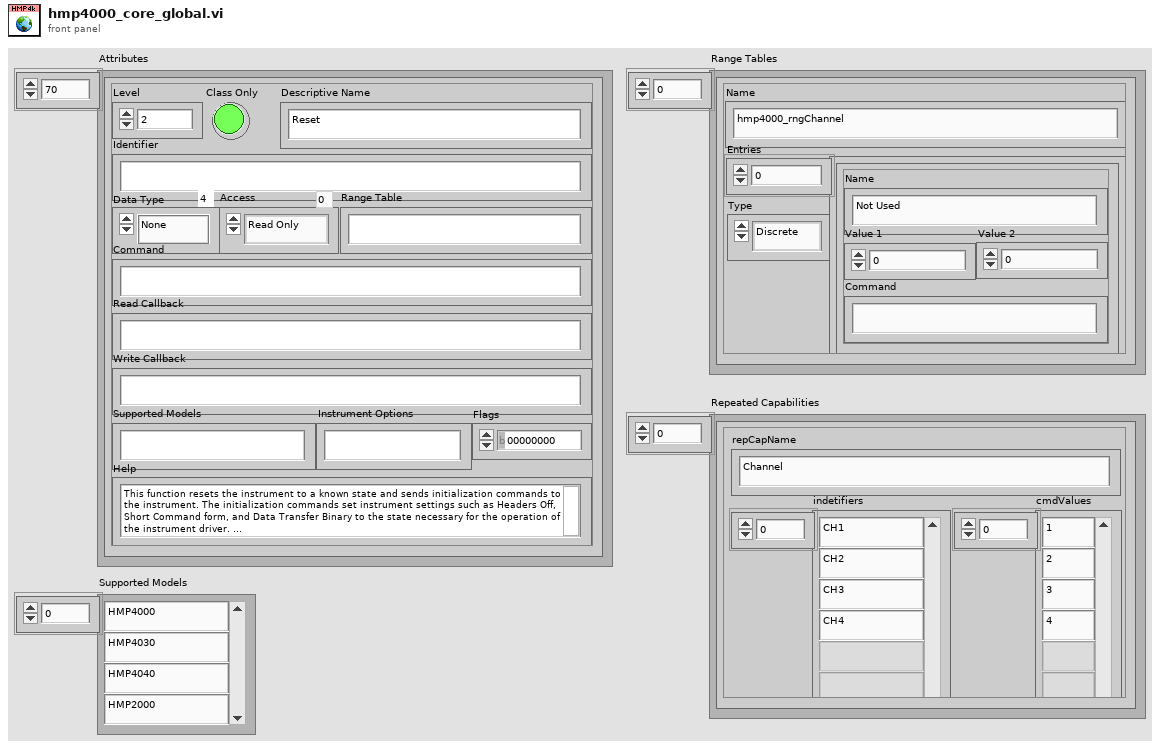
[diagram p1: front panel]
types:
  T1 = typedef "hmp4000_rsidr_core.lvlib/type_Input_Format_RepCap.ctl" = cluster{"repCapName":string, "indetifiers":string[], "cmdValues":string[]}
  T2 = typedef "hmp4000_rsidr_core.lvlib/type_Input_Format_RangeTable.ctl" = cluster{"Type":u16, "Name":string, "Entries":cluster{"Name":string, "Value 1":dbl, "Value 2":dbl, "Command":string}[]}
  T3 = typedef "hmp4000_rsidr_core.lvlib/type_Input_Format_Attribute.ctl" = cluster{"Level":i32, "Class Only":bool, "Identifier":string, "Descriptive Name":string, "Data Type":u16, "Command":string, "Access":u16, "Range Table":string, "Read Callback":string, "Write Callback":string, "Supported Models":string, "Instrument Options":string, "Flags":i32, "Help":string}
diagram:
